vi "Alt_Alpha_Ver 1.1.vi"() -> ()   [LabVIEW 2015]
uses:
  <instrlib>/Keithley 622x LV 2009/Configure/Units/Typedefs/KE622x -- Voltage Meas Units.ctl
  <instrlib>/Keithley 622x LV 2009/Configure/2182 -A/Low Level/Typedefs/KE2182 -- Voltage Ranges.ctl
  <instrlib>/Keithley 622x LV 2009/Configure/2182 -A/Low Level/Typedefs/KE2182 -- Filter Type.ctl
  <instrlib>/Keithley 622x LV 2009/Configure/2182 -A/Low Level/Typedefs/KE2182 -- Filter Count.ctl
  <instrlib>/Keithley 622x LV 2009/Configure/2182 -A/Low Level/Typedefs/KE2182 -- Filter Window.ctl
  <instrlib>/Keithley 622x LV 2009/Configure/2182 -A/Low Level/Typedefs/KE2182 -- NPLCs.ctl
  <instrlib>/Keithley 622x LV 2009/Configure/Units/Typedefs/KE6221 -- PDelta Power Meas Type.ctl
  <instrlib>/Keithley 622x LV 2009/Configure/Delta PDelta DCon Modes/Typedefs/KE6221 -- PDelta Mode Params.ctl
  <instrlib>/Keithley 622x LV 2009/Configure/Delta PDelta DCon Modes/Low Level/Typedefs/KE622x -- Delta PDelta Mode High Level.ctl
  <instrlib>/Keithley 622x LV 2009/Configure/Delta PDelta DCon Modes/Low Level/Typedefs/KE622x -- Delta PDelta Mode Low Level.ctl
  <instrlib>/Keithley 622x LV 2009/Configure/Delta PDelta DCon Modes/Low Level/Typedefs/KE6221 -- PDelta Mode Pulse Width.ctl
  <instrlib>/Keithley 622x LV 2009/Configure/Delta PDelta DCon Modes/Low Level/Typedefs/KE6221 -- PDelta Mode Source Delay.ctl
  <instrlib>/Keithley 622x LV 2009/Configure/Delta PDelta DCon Modes/Low Level/Typedefs/KE622x -- Delta PDelta Mode Num Cycles Mode.ctl
  <instrlib>/Keithley 622x LV 2009/Configure/Delta PDelta DCon Modes/Low Level/Typedefs/KE622x -- Delta PDelta Mode Num Cycles.ctl
  <instrlib>/Keithley 622x LV 2009/Configure/Delta PDelta DCon Modes/Low Level/Typedefs/KE6221 -- PDelta Mode Ranging Mode.ctl
  <instrlib>/Keithley 622x LV 2009/Configure/Delta PDelta DCon Modes/Low Level/Typedefs/KE6221 -- PDelta Mode Num Low Meas.ctl
  <instrlib>/Keithley 622x LV 2009/Configure/Delta PDelta DCon Modes/Low Level/Typedefs/KE6221 -- PDelta Mode Pulse Period.ctl
  <instrlib>/Keithley 622x LV 2009/Configure/Format/Typedefs/KE622x -- Optional Meas Elements.ctl
  <instrlib>/Keithley 622x LV 2009/Configure/Trace Buf/Low Level/Typedefs/KE622x -- Trace Buf.ctl
  <instrlib>/Keithley 622x LV 2009/Utility/Typedefs/KE622x -- Instrument Type.ctl
  <instrlib>/Keithley 622x LV 2009/Keithley 622x.lvlib
panel:
  out "Trace Buf":T1 {"Average Voltage (V)" format="%.3p"; "Source Val (A)" format="%.3p"; "Timestamp (secs)" format="%.3f"; "Reading" format="%.3p"}
  in  "Meas Elements To Return":T2={"Timstamp?"=TRUE, "Reading Num?"=TRUE, "Source Value?"=FALSE, "Compliance?"=FALSE, "Average Voltage?"=FALSE}
  in  "stop":bool
  in  "Check For SCPI Errors? (T)":bool=TRUE
  in  "Power Meas Type":T3
  in  "2812 -A Params In":T9={"Auto Range?"=FALSE, "Man / Selected\nRange"=enum."10mV", "Enable Digital\nFilter?"=FALSE, "Filter Type"=enum."Moving", "Filter Count"=10, "Filter\nWindow (%)"=0.01, "Enable Analog\nFilter?"=FALSE, "NPLCs"=5} {"Filter\nWindow (%)" min=0.0 max=10.0 step=0.01 format="%.2f"; "Filter Count" min=1 max=100; "NPLCs" min=1 max=10}
  in  "Measurement Units":T10
  in  "Measurements control":enum32{"PULSE", " DELTA"}(tab)
  in  "Pulsed Delta Mode Params In":T11={"High Level (A)"=0.001, "Low Level (A)"=0.0, "Pulse Width (s)"=0.00011, "Source Delay (s)"=1.6e-05, "Num Cycles Mode"=enum."Finite Count", "Finite Count"=1, "Ranging Mode"=enum."Best", "Num Low Meas Per Cycle"=enum."1", "Pulse Period (Num PLCs)"=5, "Pulse Sweep Mode Enabled?"=FALSE} {"Pulse Period (Num PLCs)" min=5 max=999990; "Source Delay (s)" min=1.6e-05 max=0.011966 format="%.3p"; "Pulse Width (s)" min=5e-05 max=0.012 format="%.3p"; "Finite Count" min=2 max=65536; "Low Level (A)" min=-0.105 max=0.0 format="%.3p"; "High Level (A)" min=0.0 max=0.105 format="%.3p"}
  in  "Comments":string
  in  "Folder \nPrename":string
  # "Keithley  6221 & 2182A Measurement System"
  # "FILE CONFIGURATION"
  # "PRE EXPERIMENT CONFIGS"
  # "*** NOTE:  \"Average Voltage\"\nis only available for Differential\nConductance measurements."
  # "*** NOTE:  \"Average Voltage\"\nis only available for Differential\nConductance measurements."
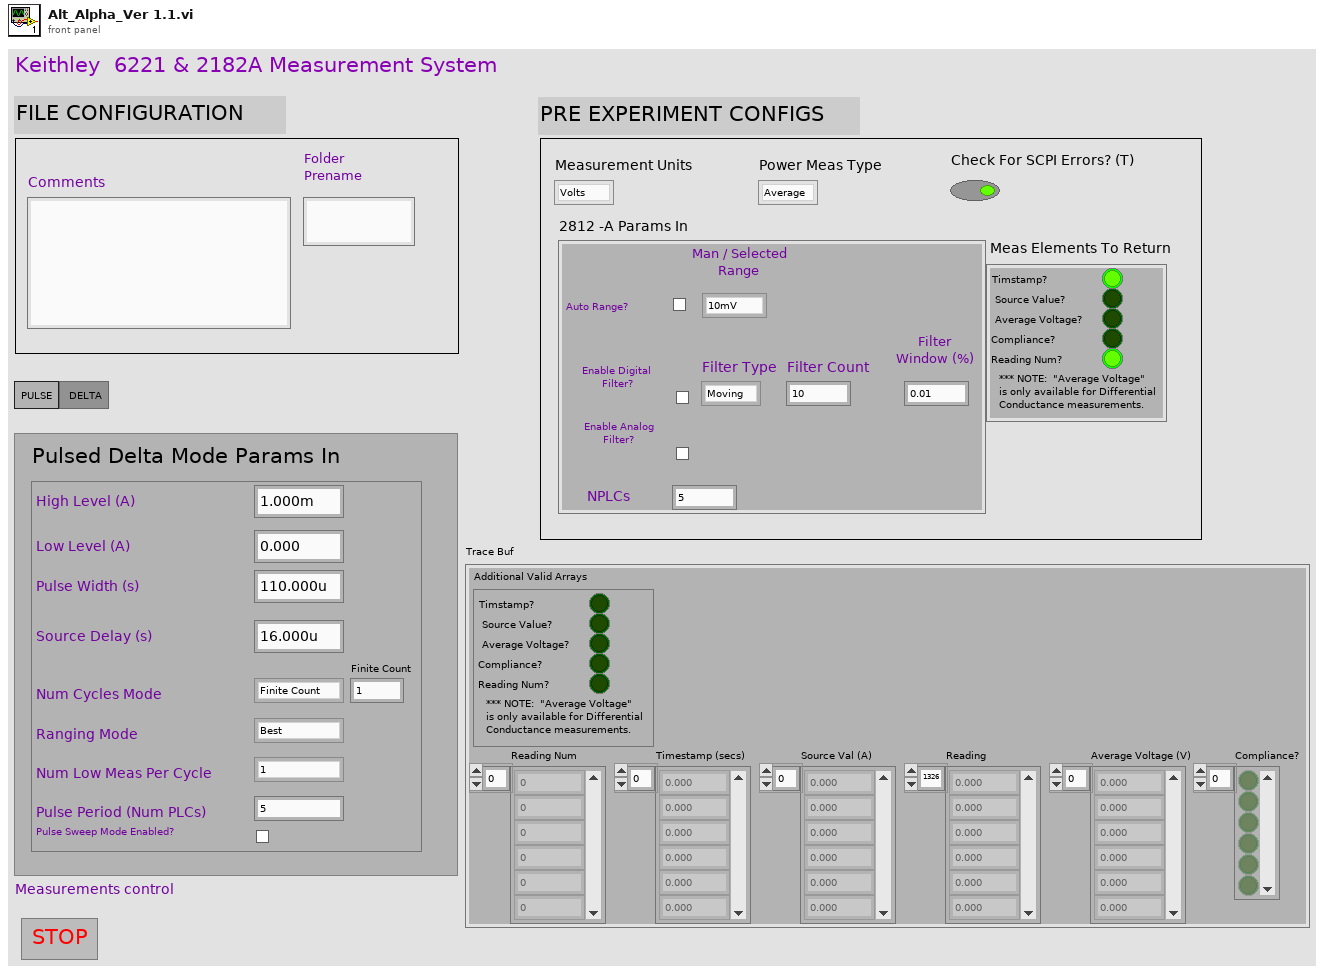
[diagram p1: front panel]
types:
  T1 = typedef "Keithley 622x.lvlib/KE622x -- Trace Buf.ctl" = cluster{"Additional Valid Arrays":T2, "Reading Num":u32[], "Timestamp (secs)":sgl[], "Source Val (A)":sgl[], "Reading":sgl[], "Average Voltage (V)":sgl[], "Compliance?":bool[]}
  T2 = typedef "Keithley 622x.lvlib/KE622x -- Optional Meas Elements.ctl" = cluster{"Timstamp?":bool, "Reading Num?":bool, "Source Value?":bool, "Compliance?":bool, "Average Voltage?":bool}
  T3 = typedef "Keithley 622x.lvlib/KE6221 -- PDelta Power Meas Type.ctl" = enum16{"Average", "Peak"}
  T4 = typedef "Keithley 622x.lvlib/KE2182 -- Voltage Ranges.ctl" = enum16{"10mV", "100mV", "1V", "10V", "100V"}
  T5 = typedef "Keithley 622x.lvlib/KE2182 -- Filter Type.ctl" = enum16{"Moving", "Repeat"}
  T6 = typedef "Keithley 622x.lvlib/KE2182 -- Filter Count.ctl" = u32
  T7 = typedef "Keithley 622x.lvlib/KE2182 -- Filter Window.ctl" = dbl
  T8 = typedef "Keithley 622x.lvlib/KE2182 -- NPLCs.ctl" = u32
  T9 = cluster{"Auto Range?":bool, "Man / Selected\nRange":T4, "Enable Digital\nFilter?":bool, "Filter Type":T5, "Filter Count":T6, "Filter\nWindow (%)":T7, "Enable Analog\nFilter?":bool, "NPLCs":T8}
  T10 = typedef "Keithley 622x.lvlib/KE622x -- Voltage Meas Units.ctl" = enum16{"Volts", "Ohms", "Watts", "Siemens"}
  T11 = typedef "Keithley 622x.lvlib/KE6221 -- PDelta Mode Params.ctl" = cluster{"High Level (A)":T12, "Low Level (A)":T13, "Pulse Width (s)":T14, "Source Delay (s)":T15, "Num Cycles Mode":T16, "Finite Count":T17, "Ranging Mode":T18, "Num Low Meas Per Cycle":T19, "Pulse Period (Num PLCs)":T20, "Pulse Sweep Mode Enabled?":bool}
  T12 = typedef "Keithley 622x.lvlib/KE622x -- Delta PDelta Mode High Level.ctl" = dbl
  T13 = typedef "Keithley 622x.lvlib/KE622x -- Delta PDelta Mode Low Level.ctl" = dbl
  T14 = typedef "Keithley 622x.lvlib/KE6221 -- PDelta Mode Pulse Width.ctl" = dbl
  T15 = typedef "Keithley 622x.lvlib/KE6221 -- PDelta Mode Source Delay.ctl" = dbl
  T16 = typedef "Keithley 622x.lvlib/KE622x -- Delta PDelta Mode Num Cycles Mode.ctl" = enum16{"Finite Count", "Infinite"}
  T17 = typedef "Keithley 622x.lvlib/KE622x -- Delta PDelta Mode Num Cycles.ctl" = u32
  T18 = typedef "Keithley 622x.lvlib/KE6221 -- PDelta Mode Ranging Mode.ctl" = enum16{"Best", "Fixed"}
  T19 = typedef "Keithley 622x.lvlib/KE6221 -- PDelta Mode Num Low Meas.ctl" = enum16{"1", "2"}
  T20 = typedef "Keithley 622x.lvlib/KE6221 -- PDelta Mode Pulse Period.ctl" = u32
  T21 = typedef "Keithley 622x.lvlib/KE622x -- Instrument Type.ctl" = enum16{"KE6220", "KE6221"}
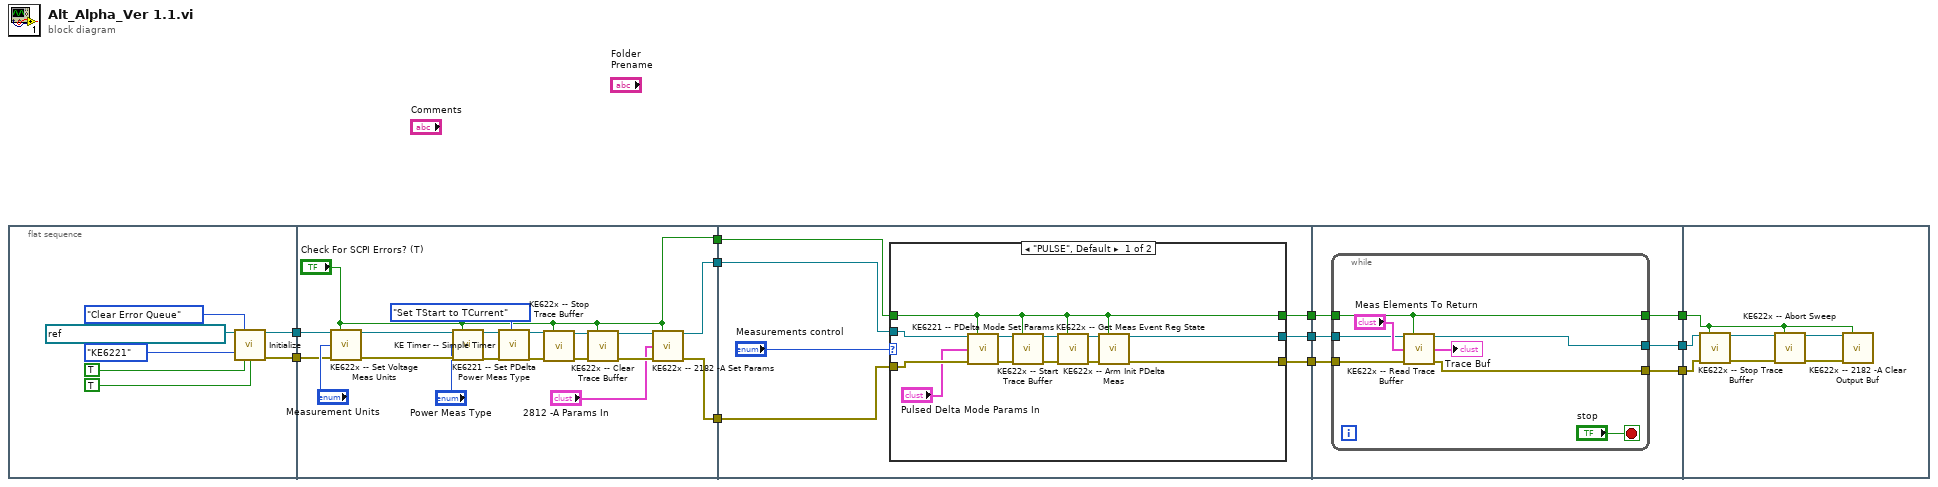
[diagram p0: block diagram]
diagram:
  n1 = flat-sequence {
    tunnel: [w13] -> w11
    tunnel: [w12] -> w10
    tunnel: w11 -> [w36]
    tunnel: w10 -> [w35]
    tunnel: [w26] -> w9
    tunnel: [w25] -> w8
    tunnel: ["Check For SCPI Errors? (T)"] -> w7
    tunnel: w9 -> [w42]
    tunnel: w8 -> [w43]
    tunnel: w7 -> [w41]
    tunnel: [w40] -> w6
    tunnel: [w39] -> w5
    tunnel: [w38] -> w4
    tunnel: w6 -> [w65]
    tunnel: w5 -> [w64]
    tunnel: w4 -> [w63]
    tunnel: [w62] -> w3
    tunnel: [w61] -> w2
    tunnel: [w60] -> w1
    tunnel: w3 -> [w76]
    tunnel: w2 -> [w75]
    tunnel: w1 -> [w74]
    frame #0 {
      n2 = call <instrlib>:"Initialize.vi"("VISA resource name"=refnum<visa-resource-name> "DC_AC_Current_Source_6221", "Error Queue Option"=enum16{"Clear Error Queue", "Error Query"}."Clear Error Queue", "Instrument Type"=KE622x_--_Instrument_Type."KE6221", "ID Query? (T)"=TRUE, "Reset? (T)"=TRUE) -> ("VISA resource name out"=w13:refnum<visa-resource-name>, "error out"=w12:errorcluster)  [unwired: 9 in]
    }
    frame #1 {
      n3 = call <instrlib>:"KE622x -- Set Voltage Meas Units.vi"("Resource In"=w36, "Check For SCPI Errors? (T)"="Check For SCPI Errors? (T)", "Voltage Meas Units"="Measurement Units", "error in (no error)"=w35) -> ("Resource Out (dupl)"=w24:refnum<visa-resource-name>, "error out"=w23:errorcluster)  [unwired: 10 in]
      n4 = call <instrlib>:"KE6221 -- Set PDelta Power Meas Type.vi"("6221 Resource In"=w24, "Check For SCPI Errors? (T)"="Check For SCPI Errors? (T)", "Power Meas Type"="Power Meas Type", "error in (no error)"=w23) -> ("6221 Resource Out (dupl)"=w21:refnum<visa-resource-name>, "error out"=w20:errorcluster)  [unwired: 10 in]
      n5 = call <instrlib>:"KE Timer -- Simple Timer.vi"("Resource In"=w21, "error in (no error)"=w20, "Action"=enum16{"Set TStart to TCurrent", "Get Deltas"}."Set TStart to TCurrent") -> ("Resource Out (dupl)"=w33:refnum<visa-resource-name>, "error out (dupl)"=w32:errorcluster)  [unwired: 7 in, 8 out]
      n6 = call <instrlib>:"KE622x -- Stop Trace Buffer.vi"("Resource In"=w33, "Check For SCPI Errors? (T)"="Check For SCPI Errors? (T)", "error in (no error)"=w32) -> ("Resource Out (dupl)"=w31:refnum<visa-resource-name>, "error out"=w30:errorcluster)  [unwired: 11 in]
      n7 = call <instrlib>:"KE622x -- Clear Trace Buffer.vi"("Resource In"=w31, "Check For SCPI Errors? (T)"="Check For SCPI Errors? (T)", "error in (no error)"=w30) -> ("Resource Out (dupl)"=w29:refnum<visa-resource-name>, "error out"=w28:errorcluster)  [unwired: 11 in]
      n8 = call <instrlib>:"KE622x -- 2182 -A Set Params.vi"("622x Resource In"=w29, "Check For SCPI Errors? (T)"="Check For SCPI Errors? (T)", "2812 -A Params In"="2812 -A Params In", "error in (no error)"=w28) -> ("622x Resource Out (dupl)"=w26:refnum<visa-resource-name>, "error out"=w25:errorcluster)  [unwired: 9 in, 1 out]
    }
    frame #2 {
      n9 = case shown="\"PULSE\", Default" "Measurements control" {
        tunnel: w43 -> [w55 w58]
        tunnel: w42 -> [w56 w59]
        tunnel: w41 -> [w45 w57]
        tunnel: [w47 w59] -> w40
        tunnel: [w46 w58] -> w39
        tunnel: [w45 w57] -> w38
        frame "PULSE", Default {
          n10 = call <instrlib>:"KE6221 -- PDelta Mode Set Params.vi"("6221 Resource In"=w56, "Check For SCPI Errors? (T)"=w45, "Pulsed Delta Mode Params In"="Pulsed Delta Mode Params In", "error in (no error)"=w55) -> ("6221 Resource Out (dupl)"=w53:refnum<visa-resource-name>, "error out"=w52:errorcluster)  [unwired: 9 in, 1 out]
          n11 = call <instrlib>:"KE622x -- Start Trace Buffer.vi"("Resource In"=w53, "Check For SCPI Errors? (T)"=w45, "error in (no error)"=w52) -> ("Resource Out (dupl)"=w51:refnum<visa-resource-name>, "error out"=w50:errorcluster)  [unwired: 11 in]
          n12 = call <instrlib>:"KE622x -- Get Meas Event Reg State.vi"("VISA Resource In"=w51, "Error Query (T)?"=w45, "error in (no error)"=w50) -> ("VISA Resource Out (dupl)"=w49:refnum<visa-resource-name>, "error out"=w48:errorcluster)  [unwired: 10 in, 1 out]
          n13 = call <instrlib>:"KE622x -- Arm Init PDelta Meas.vi"("Resource In"=w49, "Check For SCPI Errors? (T)"=w45, "error in (no error)"=w48) -> ("Resource Out (dupl)"=w47:refnum<visa-resource-name>, "error out"=w46:errorcluster)  [unwired: 11 in]
        }
        frame " DELTA" {
        }
      }
    }
    frame #3 {
      n14 = while {
        tunnel: w65 -> [w70]
        tunnel: w64 -> [w71]
        tunnel: w63 -> [w68]
        tunnel: [w68] -> w62
        tunnel: [w67] -> w61
        tunnel: [w66] -> w60
        stop <- "stop" stop-if-true
        n15 = call <instrlib>:"KE622x -- Read Trace Buffer.vi"("Resource In"=w70, "Check For SCPI Errors? (T)"=w68, "Meas Elements To Return"="Meas Elements To Return", "error in (no error)"=w71) -> ("Resource Out (dupl)"=w67:refnum<visa-resource-name>, "Trace Buf"=→"Trace Buf":T1, "error out"=w66:errorcluster)  [unwired: 9 in]
      }
    }
    frame #4 {
      n16 = call <instrlib>:"KE622x -- Stop Trace Buffer.vi"("Resource In"=w75, "Check For SCPI Errors? (T)"=w76, "error in (no error)"=w74) -> ("Resource Out (dupl)"=w80:refnum<visa-resource-name>, "error out"=w78:errorcluster)  [unwired: 11 in]
      n17 = call <instrlib>:"KE622x -- Abort Sweep.vi"("Resource In"=w80, "Check For SCPI Errors? (T)"=w76, "error in (no error)"=w78) -> ("Resource Out (dupl)"=w79:refnum<visa-resource-name>, "error out"=w77:errorcluster)  [unwired: 11 in]
      n18 = call <instrlib>:"KE622x -- 2182 -A Clear Output Buf.vi"("622x Resource In"=w79, "Check For SCPI Errors? (T)"=w76, "error in (no error)"=w77) -> ()  [unwired: 10 in, 3 out]
    }
  }
